vi "34401A Multi_point.vi"(0 "VISA resource name":refnum<visa-resource-name>, 2 "Timeout":i32=10000, 7 "Function (0: DC Voltage)":u16(ring) items=["DC Voltage", "AC Voltage", "2 - Wire Resistance", "4 - Wire Resistance", "DC Current", "AC Current", "Frequency", "Period", "Continuity", "Diode Checking", "VDC:VDC Ratio", "Temperature", "Capacitance"], 9 "Sample Count (10)":i32=10, 11 "error in (no error)":errorcluster) -> (4 "mean":dbl format="%0.3e", 8 "Measurements":dbl[](array[numeric]) format="%#_8g", 10 "status":bool, 15 "error out":errorcluster)   [LabVIEW 2019]
uses:
  <vilib>/Analysis/baseanly.llb/Mean (DBL).vi
  <userlib>/_TI-LA/Instr Drivers/Multimeter/34401A/Driver/Base/Public/Data/Read (Single Point).vi
  <userlib>/_TI-LA/Instr Drivers/Multimeter/34401A/Driver/34401A.lvlib
  <vilib>/Analysis/NI_AALBase.lvlib
panel:
  in  "Set":bool=TRUE
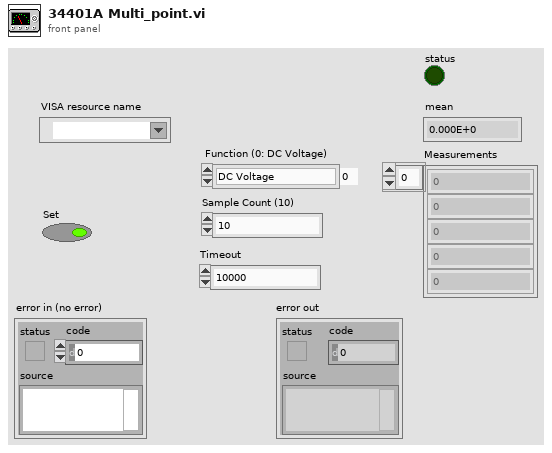
[diagram p1: front panel]
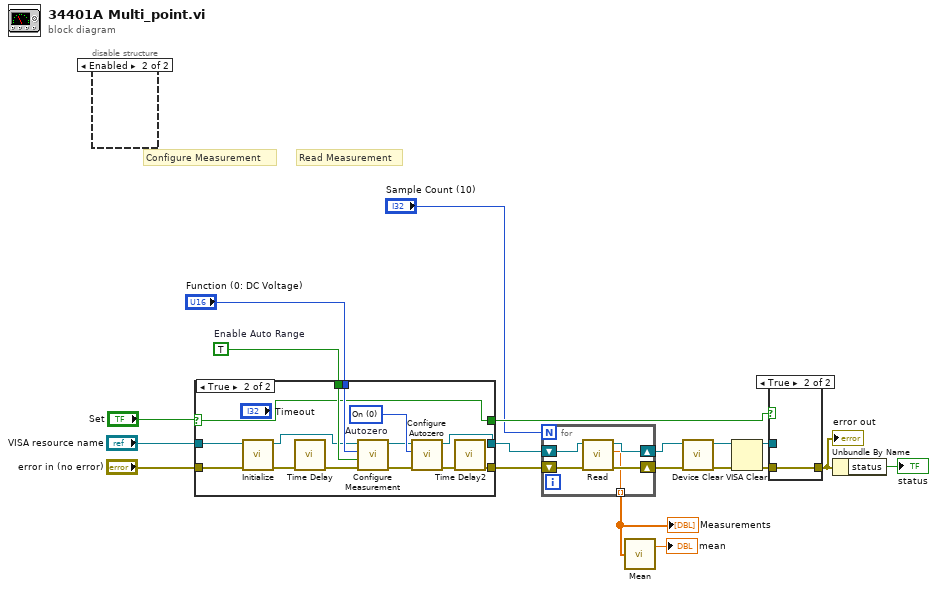
[diagram p0: block diagram]
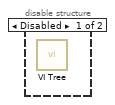
[diagram p4: hidden frame]
diagram:
  w15 = TRUE  # Enable Auto Range
  # "Read Measurement"
  # "Configure Measurement"
  n1 = disable-structure shown="Enabled" {
    frame Disabled {
      n2 = call <userlib>:"VI Tree.vi"() -> ()  [unwired: 12 in]
    }
    frame Enabled {
    }
  }
  n3 = case shown="True" "Set" {
    selector: "Set" -> [w20 w23]
    tunnel: "error in (no error)" -> [w21 w36]
    tunnel: "Function (0: DC Voltage)" -> [_ w35]
    tunnel: [w22 w34] -> w16
    tunnel: w15 -> [_ w30]
    tunnel: "VISA resource name" -> [w22 w28]
    tunnel: [w21 w24] -> w9
    tunnel: [w20 w23] -> w3
    frame False {
    }
    frame True {
      w33 = u16 0 items=["On", "Off", "Once"]  # Autozero
      n4 = call <userlib>:"Initialize.vi"("error in (no error)"=w36, "VISA resource name"=w28) -> ("error out"=w27:errorcluster, "VISA resource name out"=w29:refnum<visa-resource-name>)  [unwired: 8 in]
      n5 = call "Time Delay"("error in (no error)"=w27) -> ("error out"=w26:errorcluster)  [unwired: 10 in]
      n6 = call <userlib>:"Configure Measurement.vi"("error in (no error)"=w26, "Enable Auto Range (T: Enable)"=w30, "Function (0: DC Voltage)"=w35, "VISA resource name"=w29) -> ("error out"=w31:errorcluster, "VISA resource name out"=w32:refnum<visa-resource-name>)  [unwired: 6 in]
      n7 = call <userlib>:"Configure Autozero.vi"("error in (no error)"=w31, "Autozero  (0: On)"=w33, "VISA resource name"=w32) -> ("error out"=w25:errorcluster, "VISA resource name out"=w34:refnum<visa-resource-name>)  [unwired: 7 in]
      n8 = call "Time Delay2"("error in (no error)"=w25) -> ("error out"=w24:errorcluster)  [unwired: 10 in]
    }
  }
  n9 = for {
    N: "Sample Count (10)" -> [_]
    shift-right: [w40] -> w12
    shift-left: w16 -> [w41]
    shift-right: [w39] -> w11
    shift-left: w9 -> [w38]
    tunnel: [w37] -> w1 mode=indexing
    n10 = call-poly <userlib>:"Read.vi"("error in (no error)"=w38, "VISA resource name"=w41) -> ("error out"=w39:errorcluster, "Measurement"=w37:dbl, "VISA resource name out"=w40:refnum<visa-resource-name>)  [unwired: 7 in]
  }
  "Measurements" <- w1
  n11 = call-poly <vilib>:"Mean.vi"("X"=w1) -> ("mean"=→"mean":dbl)  [unwired: 1 out]
  n12 = call <userlib>:"Device Clear.vi"("error in (no error)"=w11, "VISA Resource Name"=w12) -> ("error out"=w7:errorcluster, "VISA Resource Out"=w8:refnum<visa-resource-name>)  [unwired: 8 in]
  n13 = VISA Clear(VISA resource name=w8, error in (no error)=w7) -> (VISA resource name out=w6:refnum<visa-resource-name>, error out=w5:errorcluster)
  n14 = case shown="True" w3 {
    tunnel: [w42 w43] -> w10
    tunnel: w6 -> [_ _]
    tunnel: w5 -> [w42 w43]
    frame False {
    }
    frame True {
    }
  }
  "error out" <- w10
  n15 = Unbundle By Name(w10) -> ("status"=→"status":bool)
